vi "WriteAppDataToFile.vi"(8 "ErrorArray In":errorcluster[](array[cluster]), 10 "Bus.lvclass In":refnum<class "Bus.lvclass">, 11 "TestFileRef In":T1) -> (0 "ErrorArray Out":errorcluster[](array[cluster]), 2 "Bus.lvclass Out":refnum<class "Bus.lvclass">, 3 "TestFileRef Out":T1)   [LabVIEW 2014, in "Bus_class.lvlib" / "Bus.lvclass"]
uses:
  Bus.lvclass
  <vilib>/Utility/config.llb/Config Data RefNum.ctl
  TypeDefs/clBusData.ctl
  FrontPanel/TypeDefs/clEventConfig.ctl
  Modules/PmuImpairPlugins/PmuImpairPluginBase_class/TypeDefs/clImpairConfig.ctl
  Modules/EventPlugins/EventPluginBaseClass/TypeDefs/clEvtReportArray.ctl
  Modules/EventPlugins/EventPluginBaseClass/TypeDefs/clEvtReport.ctl
  Modules/EventPlugins/EventPluginBaseClass/TypeDefs/dblEvtSignalArray.ctl
  Modules/NetworkImpairmentModule/PublicAPI/Arguments/Broadcasts/dblNetworkTime.ctl
  Modules/NetworkImpairmentModule/PublicAPI/Arguments/Broadcasts/dblPktLoss.ctl
  Modules/FlagImpairModule/PublicAPI/Arguments/Broadcasts/ui32FlagImpairmentArray.ctl
  Modules/OutputToFilePlugins/OutputToFileBasePlugin/Typedefs/PmuCfgOpt.ctl
  Modules/AppModule/AppModule.lvlib
  <userlib>/NIST/NISTErrorLib/NISTErrorLib.lvlib
  <vilib>/ErrorRing/Error Ring.xnode
  <vilib>/Utility/error.llb/Error Cluster From Error Code.vi
  Modules/EventModule/PublicAPI/Arguments/Broadcasts/clErrorRpt.ctl
  Modules/EventModule/EventModule.lvlib
  Framework.lvlib
  Modules/PmuImpairPlugins/PmuImpairPluginBase_class/PmuImpairPluginBase.lvclass
  Modules/EventPlugins/EventPluginBaseClass/EventPluginBaseClass.lvclass
  Modules/NetworkImpairmentModule/NetworkImpairmentModule.lvlib
  Modules/FlagImpairModule/FlagImpairModule.lvlib
  Modules/OutputToFilePlugins/OutputToFileBasePlugin/OutputToFileBasePlugin.lvclass
  <vilib>/Utility/config.llb/NI_LVConfig.lvlib
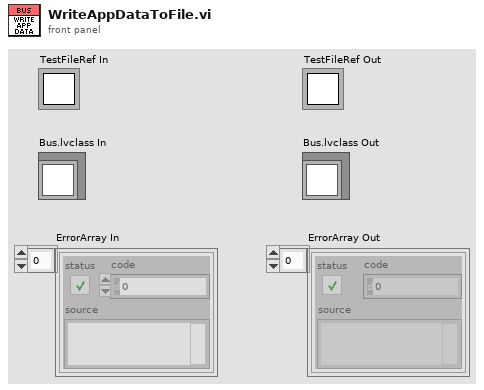
[diagram p1: front panel]
types:
  T1 = typedef "NI_LVConfig.lvlib/Config Data RefNum.ctl" = refnum<k1>
  T2 = typedef "EventModule.lvlib/clErrorRpt.ctl" = cluster{"error":errorcluster, "AdditionalInfo":string}
  T3 = typedef "Bus_class.lvlib/Bus.lvclass/clBusData.ctl" = cluster{"BusNumber":u8, "EvtPluginINIFilePath":path, "EvtParams":string[][], "EvtConfig":T4, "Start Time":dbl, "End Time":dbl, "PmuImpairPluginINIFilePath":path, "PmuImpairParams ":string[][], "PmuImpairConfig":T5, "NetImpPluginINIFilePath":path, "NetImpParams":string[][], "FlagImpPluginINIFilePath":path, "FlagImpParams":string[][], "EvtReportArray":T6, "EventSignalArray":T8, "ImpairReportArray":T6, "NetworkTime":T9, "PktLoss":T10, "FlagImpArray":T11, "OutputToFilePluginINIFilePath":path, "Output File Path":path, "clConfigOptions":T12, "AppPluginINIFilePath":path, "AppConfig":variant, "AppOutput":variant}
  T4 = typedef "Framework.lvlib/clEventConfig.ctl" = cluster{"UTC Time 0":timestamp, "Nominal Frequency":u16, "Reporting Rate":u16, "Fsamp":u32, "PosSeq":bool}
  T5 = typedef "PmuImpairPlugins.lvlib/PmuImpairPluginBase.lvclass/clImpairConfig.ctl" = cluster{"FilterType":string, "bPosSeq":bool}
  T6 = typedef "EventPlugins.lvlib/EventPluginBaseClass.lvclass/clEvtReportArray.ctl" = T7[]
  T7 = typedef "EventPlugins.lvlib/EventPluginBaseClass.lvclass/clEvtReport.ctl" = cluster{"Timestamp":dbl, "Synx":cdb[], "Freq":dbl, "ROCOF":dbl, "ID":i16}
  T8 = typedef "EventPlugins.lvlib/EventPluginBaseClass.lvclass/dblEvtSignalArray.ctl" = dbl[][]
  T9 = typedef "NetworkImpairmentModule.lvlib/dblNetworkTime.ctl" = dbl[]
  T10 = typedef "NetworkImpairmentModule.lvlib/dblPktLoss.ctl" = dbl[]
  T11 = typedef "FlagImpairModule.lvlib/ui32FlagImpairmentArray.ctl" = u32[]
  T12 = typedef "OutputToFilePlugins.lvlib/OutputToFileBasePlugin.lvclass/PmuCfgOpt.ctl" = cluster{"TIME_BASE":u64, "STN":string, "IDCODE":u16, "rdoPolRect":enum32{"Rectangular", "Polar"}, "rdoFloatInt":enum32{"Float", "Integer"}, "PHUNIT":u64, "rdoFreqDfreq":enum32{"Float", "Integer"}, "CHNAM":string[], "chkCfg2Prefix":bool}
  T13 = typedef "AppModule.lvlib/clBroadcastEvents.ctl" = cluster{"DidInit":refnum<user-event>, "StatusUpdate":refnum<user-event>, "ErrorReport":refnum<user-event>, "DidStop":refnum<user-event>, "PathToINI":refnum<user-event>, "InputData":refnum<user-event>, "OutputData":refnum<user-event>, "BcAppInfo":refnum<user-event>, "ConfigData":refnum<user-event>}
  T14 = cluster{"AppPluginIniFilePath":path, "Config":string}
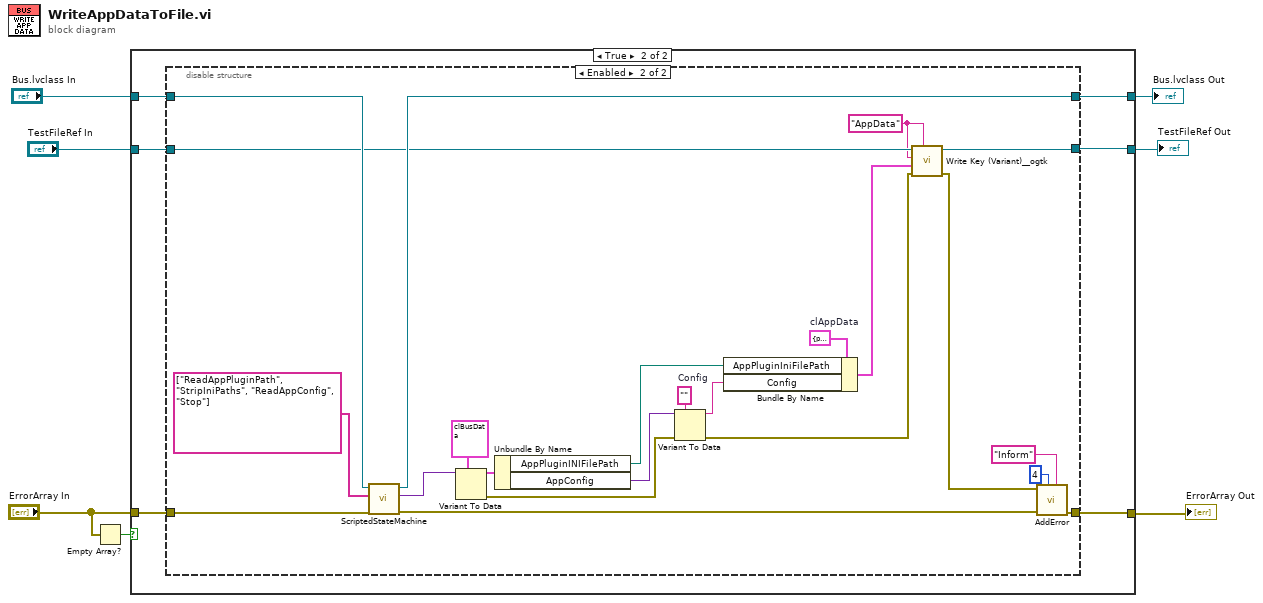
[diagram p0: block diagram]
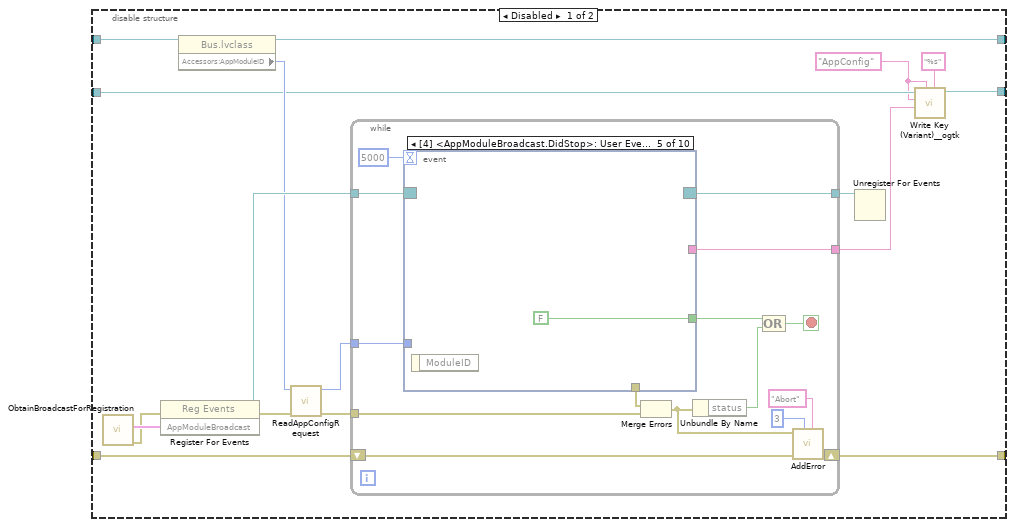
[diagram p3: hidden frame]
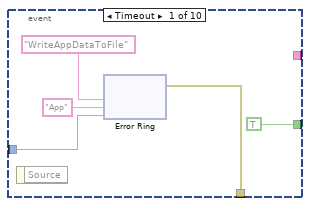
[diagram p4: hidden frame]
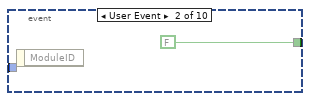
[diagram p5: hidden frame]
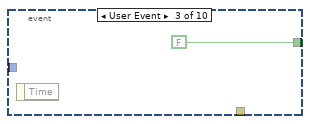
[diagram p6: hidden frame]
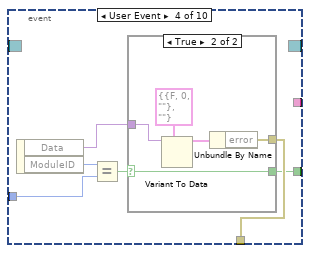
[diagram p7: hidden frame]
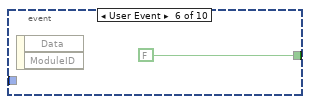
[diagram p9: hidden frame]
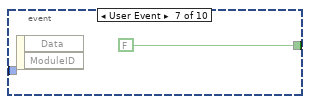
[diagram p10: hidden frame]
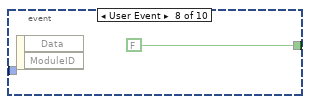
[diagram p11: hidden frame]
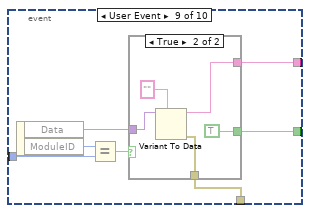
[diagram p12: hidden frame]
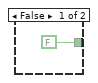
[diagram p13: hidden frame]
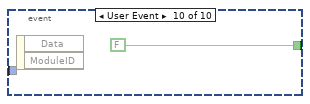
[diagram p14: hidden frame]
diagram:
  n1 = Empty Array?(array="ErrorArray In") -> (empty?=w7:bool)
  n2 = case shown="True" w7 {
    tunnel: "ErrorArray In" -> [w10 w14]
    tunnel: [w10 w13] -> w5
    tunnel: [w9 w15] -> w3
    tunnel: "Bus.lvclass In" -> [w9 w16]
    tunnel: [w8 w12] -> w1
    tunnel: "TestFileRef In" -> [w8 w11]
    frame False {
    }
    frame True {
      n3 = disable-structure shown="Enabled" {
        disable-tunnel: w16 -> [w32 w114]
        disable-tunnel: [w24 w113] -> w15
        disable-tunnel: w14 -> [w23 w116]
        disable-tunnel: [w22 w105] -> w13
        disable-tunnel: [w21 w108] -> w12
        disable-tunnel: w11 -> [w20 w109]
        frame Disabled {
          w17 = "AppConfig" ("section")
          n4 = call "ObtainBroadcastForRegistration.vi"() -> ("error out"=w29:errorcluster, "AppModuleBroadcast"=w31:T13)  [unwired: 10 in]
          n5 = register-events(error in=w29, w31) -> (reference out=w30:refnum<event-registration>, error out=w28:errorcluster)  [unwired: 1 in]
          n6 = property class="Bus.lvclass"(reference=w32) -> (reference out=w24:refnum<class "Bus.lvclass">, "Accessors:AppModuleID"=w27:i32)  [unwired: 1 in, 1 out]
          n7 = call "ReadAppConfigRequest.vi"("error in (no error)"=w28, "ModuleID"=w27) -> ("error out"=w25:errorcluster)  [unwired: 9 in]
          n8 = while {
            tunnel: w27 -> [w46]
            tunnel: w30 -> [w45]
            shift-right: [w43] -> w22
            shift-left: w23 -> [w44]
            tunnel: [w39] -> w26
            tunnel: w25 -> [w35]
            tunnel: [w33] -> w18
            stop <- w40 stop-if-true
            n9 = event shown="[4] <AppModuleBroadcast.DidStop>: User Event" {
              selector: w45 -> [_ _ _ _ _ _ _ _ _ _]
              dyn-events: [_ _ _ _ _ _ _ _ _ _] -> w39
              timeout: 5000 -> [_ _ _ _ _ _ _ _ _ _]
              tunnel: w46 -> [w49 _ _ w69 _ _ _ _ w85 _]
              tunnel: [w52 _ _ w66 _ _ _ _ w81 _] -> w36
              tunnel: [TRUE FALSE FALSE w64 FALSE FALSE FALSE FALSE w83 FALSE] -> w42
              tunnel: [_ _ _ _ _ _ _ _ w80 _] -> w33
              event Timeout {
                n10 = event-data() -> ()  [unwired: 1 in, 1 out]
                n11 = xnode "Error Ring"("parameter 0"="WriteAppDataToFile" ("ScriptCmd"), "parameter 1"="App" ("parameter 0"), "parameter 2"=w49) -> ("error out"=w52:errorcluster)
              }
              event User Event {
                n12 = event-data() -> ()  [unwired: 1 in, 1 out]
              }
              event User Event {
                n13 = event-data() -> ()  [unwired: 1 in, 1 out]
              }
              event User Event {
                n14 = event-data() -> ("Data"=w67:variant, "ModuleID"=w68:i32)  [unwired: 1 in]
                n15 = Equal?(x=w68, y=w69) -> (x = y?=w65:bool)
                n16 = case shown="True" w65 {
                  selector: w65 -> [w70 w71]
                  tunnel: w67 -> [_ w75]
                  tunnel: [_ w72] -> w66
                  tunnel: [w70 w71] -> w64
                  frame False {
                  }
                  frame True {
                    n17 = Variant To Data(type=T2 {"error"={"status"=FALSE, "code"=0, "source"=""}, "AdditionalInfo"=""} ("Cluster"), Variant=w75) -> (data=w73:T2)  [unwired: 1 in, 1 out]
                    n18 = Unbundle By Name(w73) -> ("error"=w72:errorcluster)
                  }
                }
              }
              event User Event {
                n19 = event-data() -> ()  [unwired: 1 in, 1 out]
              }
              event User Event {
                n20 = event-data() -> ()  [unwired: 1 in, 2 out]
              }
              event User Event {
                n21 = event-data() -> ()  [unwired: 1 in, 2 out]
              }
              event User Event {
                n22 = event-data() -> ()  [unwired: 1 in, 2 out]
              }
              event User Event {
                n23 = event-data() -> ("Data"=w82:variant, "ModuleID"=w86:i32)  [unwired: 1 in]
                n24 = Equal?(x=w86, y=w85) -> (x = y?=w84:bool)
                n25 = case shown="True" w84 {
                  tunnel: [FALSE TRUE] -> w83
                  tunnel: w82 -> [_ w88]
                  tunnel: [_ w91] -> w81
                  tunnel: [_ w89] -> w80
                  frame False {
                  }
                  frame True {
                    n26 = Variant To Data(type="" ("AppPluginINIFilePath"), Variant=w88) -> (data=w89:string, error out=w91:errorcluster)  [unwired: 1 in]
                  }
                }
              }
              event User Event {
                n27 = event-data() -> ()  [unwired: 1 in, 2 out]
              }
            }
            n28 = Merge Errors(w36, w35) -> (w34:errorcluster)
            n29 = Unbundle By Name(w34) -> ("status"=w41:bool)
            n30 = Compound Arithmetic op=OR(w42, w41) -> (w40:bool)
            n31 = call <userlib>:"AddError.vi"("Severity"="Abort", "Priority"=u8 3, "ErrorArray"=w44, "error in (no error)"=w34) -> ("ErrorArray"=w43:errorcluster[])  [unwired: 6 in, 1 out]
          }
          n32 = Unregister For Events(event registration refnum=w26) -> ()  [unwired: 1 in, 1 out]
          n33 = call <userlib>:"Write Key (Variant)__ogtk.vi"("float number format"="%s", "section"=w17, "key-value"=w18, "key (optional)"=w17, "refnum"=w20) -> ("refnum out"=w21:T1)  [unwired: 5 in, 1 out]
        }
        frame Enabled {
          w94 = T14 {"AppPluginIniFilePath"=path "", "Config"=""}  # clAppData
          w100 = ""  # Config
          w95 = "AppData" ("section")
          n34 = call "ScriptedStateMachine.vi"("ErrorArray In"=w116, "Script"=string[] ["ReadAppPluginPath", "StripIniPaths", "ReadAppConfig", "Stop"], "Bus"=w114) -> ("ErrorArray Out"=w104:errorcluster[], "Data out"=w112:variant, "Bus"=w113:refnum<class "Bus.lvclass">)  [unwired: 6 in]
          n35 = Variant To Data(type=T3 {"BusNumber"=0, "EvtPluginINIFilePath"=path "", "EvtParams"=[], "EvtConfig"={"UTC Time 0"=timestamp(0 s since 1904-01-01), "Nominal Frequency"=60, "Reporting Rate"=60, "Fsamp"=960, "PosSeq"=FALSE}, "Start Time"=0.0, "End Time"=0.0, "PmuImpairPluginINIFilePath"=path "", "PmuImpairParams "=[["960"], ["8.19"], ["164"]], "PmuImpairConfig"={"FilterType"="", "bPosSeq"=TRUE}, "NetImpPluginINIFilePath"=path "", "NetImpParams"=[], "FlagImpPluginINIFilePath"=path "", "FlagImpParams"=[], "EvtReportArray"=[], "EventSignalArray"=[], "ImpairReportArray"=[], "NetworkTime"=[], "PktLoss"=[], "FlagImpArray"=[], "OutputToFilePluginINIFilePath"=path "", "Output File Path"=path "", "clConfigOptions"={"TIME_BASE"=1000000, "STN"="Bus_1", "IDCODE"=0, "rdoPolRect"=enum."Rectangular", "rdoFloatInt"=enum."Float", "PHUNIT"=1000000, "rdoFreqDfreq"=enum."Float", "CHNAM"=["VA", "VB", "VC", "V+", "IA", "IB", "IC", "I+"], "chkCfg2Prefix"=TRUE}, "AppPluginINIFilePath"=path "", "AppConfig"=variant, "AppOutput"=variant} ("clBusData"), Variant=w112) -> (data=w110:T3, error out=w97:errorcluster)  [unwired: 1 in]
          n36 = Unbundle By Name(w110) -> ("AppPluginINIFilePath"=w107:path, "AppConfig"=w99:variant)
          n37 = Variant To Data(error in=w97, type=w100, Variant=w99) -> (data=w98:string, error out=w96:errorcluster)
          n38 = Bundle By Name(cluster=w94, "AppPluginIniFilePath"=w107, "Config"=w98) -> (w106:T14)
          n39 = call <userlib>:"Write Key (Variant)__ogtk.vi"("section"=w95, "error in (no error)"=w96, "key-value"=w106, "key (optional)"=w95, "refnum"=w109) -> ("error out"=w101:errorcluster, "refnum out"=w108:T1)  [unwired: 5 in]
          n40 = call <userlib>:"AddError.vi"("Severity"="Inform", "Priority"=u8 4, "ErrorArray"=w104, "error in (no error)"=w101) -> ("ErrorArray"=w105:errorcluster[])  [unwired: 6 in, 1 out]
        }
      }
    }
  }
  "TestFileRef Out" <- w1
  "Bus.lvclass Out" <- w3
  "ErrorArray Out" <- w5
